vi "crio_FPGA_Stepper.vi"() -> ()   [LabVIEW 2019]
uses:
  <vilib>/rvi/Emulation/niFpgaSctlEmulationGetInTimedLoop.vi
  <vilib>/rvi/Emulation/niFpgaProcessEmulError.vi
  <vilib>/rvi/Emulation/niFpgaGetClockAttributes.vi
  <vilib>/rvi/Emulation/niFpgaEmulationReportErrorSimple.vi
  <vilib>/rvi/eio/common/nirviEmuTemplateMethod_errors.vi
  <vilib>/rvi/Emulation/niFpgaCriticalErrorInLSC.vi
  <vilib>/eio/EIONode/EIONode.xnode
panel:
  in  "Initial Position":i16=1
  in  "Position Control: Desired Positoin":i16=20000
  out "Controller Direction":bool
  out "Controller Enable":bool
  in  "Stepper Enable":bool
  in  "Manual Operation":bool
  in  "Rail soft limit":i16=10000
  in  "mSec to initialize a small push away from limit switch":u32=1 caption="mSec when hit limit"
  in  "mSec when hit limit":u32=100 caption="mSec to pause when hit limit"
  out "Platform Position":i16=20000
  out "Limit Switch":bool
  in  "stop":bool
  in  "Half Peirod (pulse 40MHz)":u32=10000 caption="Count(Tick) [Interval between step]"
  in  "Stepper Direction":bool
  # "1. Manual Control Mode: Turn on Manual Operation. Specify stepper direction. Hit enable to move.\n2. Auto Position Control Mode: Enter desired position. It will automatically go there.\n3. Whenever the platform hits the limit switch at the end it will reset position to 0.\n4. Rail's soft limit is only active under manual mode."
  # "Control Panel"
  # "20000 is about the limit"
  # "Every 10000 step is about 230mm,\nSo every step is about 2.3micron"
  # "High: towards limit switch,\nLow: towards NEMA"
  # "For debug"
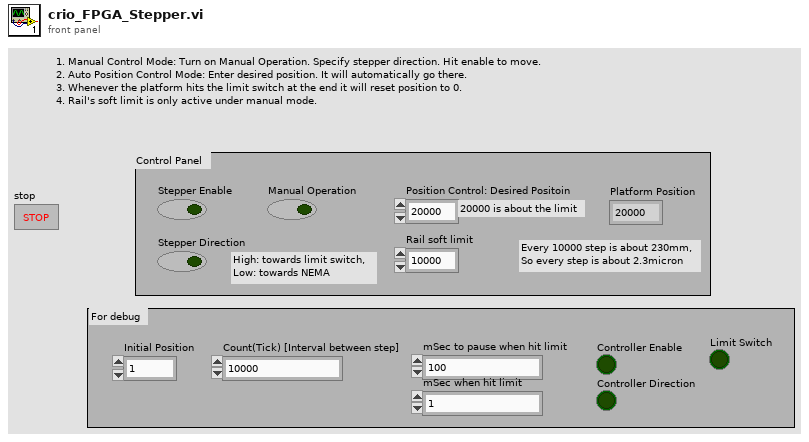
[diagram p1: front panel]
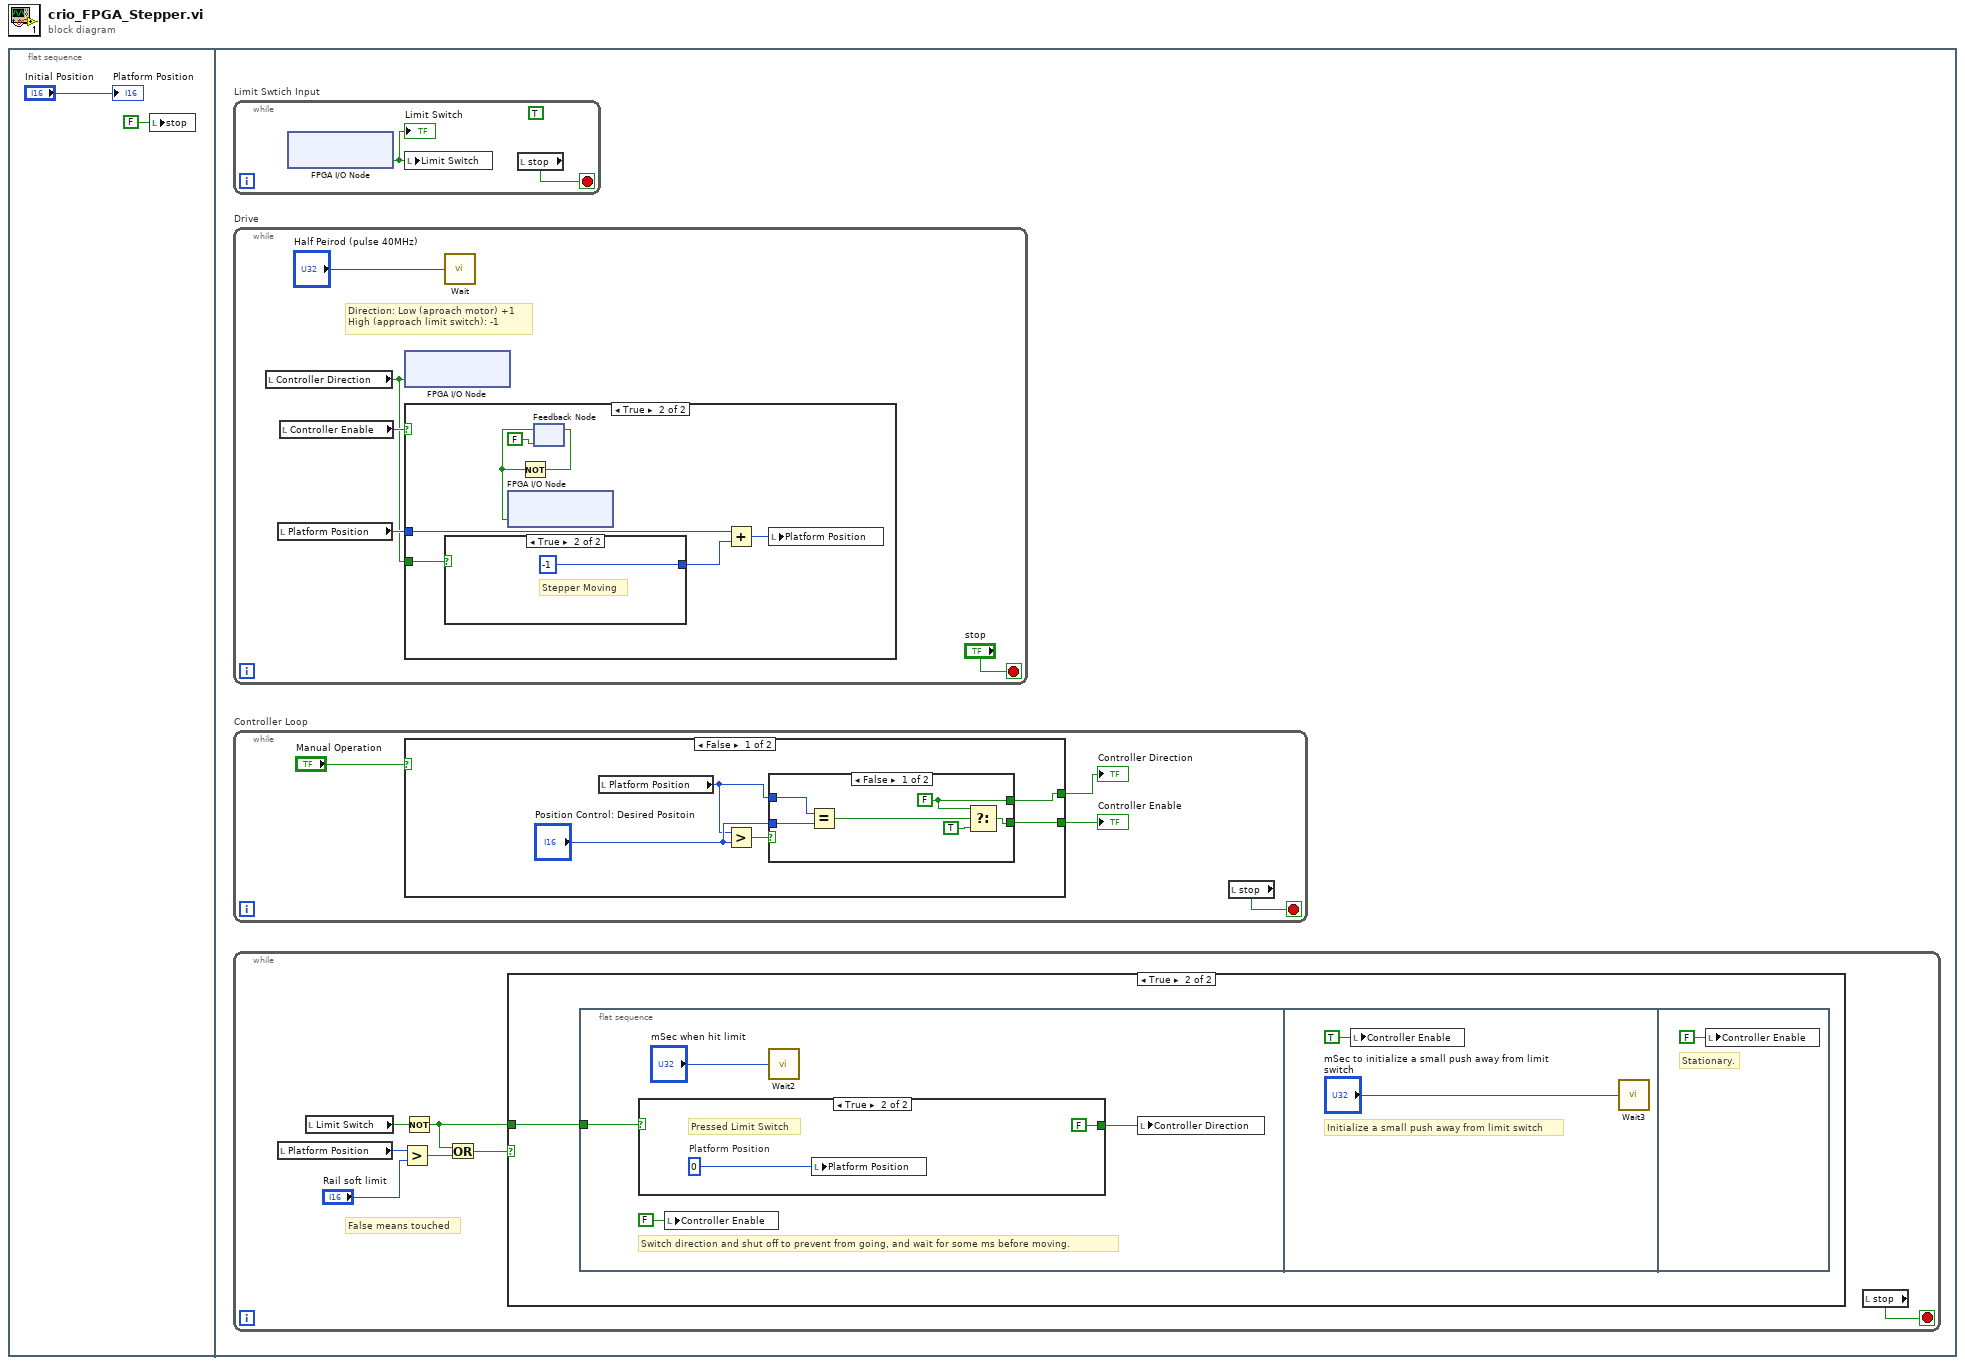
[diagram p0: block diagram]
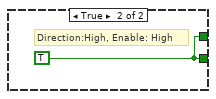
[diagram p2: hidden frame]
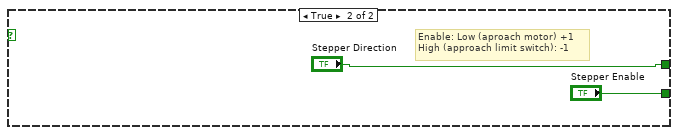
[diagram p3: hidden frame]
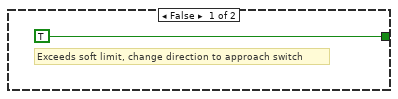
[diagram p5: hidden frame]
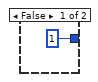
[diagram p7: hidden frame]
diagram:
  n1 = flat-sequence {
    frame #0 {
      n2 = local write "stop"(FALSE ("stop")) -> ()
      "Platform Position" <- "Initial Position"
    }
    frame #1 {
      n3 = while "Limit Swtich Input" {
        stop <- w39 stop-if-true
        (unwired) TRUE ("Mod8/DIO2")
        n4 = xnode "FPGA I/O Node"() -> ("Mod8/DIO2"=w40:bool)  [unwired: 1 in, 1 out]
        "Limit Switch" <- w40
        n5 = local write "Limit Switch"(w40) -> ()
        n6 = local read "stop"() -> (w39:bool)
      }
      n7 = while "Drive" {
        stop <- "stop" stop-if-true
        # "Direction: Low (aproach motor) +1\nHigh (approach limit switch): -1"
        n8 = local read "Controller Direction"() -> (w41:bool)
        n9 = local read "Platform Position"() -> (w43:i16)
        n10 = local read "Controller Enable"() -> (w42:bool)
        n11 = xnode "FPGA I/O Node"("Mod8/DIO4"=w41) -> ()  [unwired: 1 in, 1 out]
        n12 = case shown="True" w42 {
          tunnel: w41 -> [_ w49]
          tunnel: w43 -> [_ w46]
          frame False {
          }
          frame True {
            n13 = case shown="True" w49 {
              tunnel: [i16 1 i16 -1] -> w48
              frame False {
              }
              frame True {
                # "Stepper Moving"
              }
            }
            n14 = feedback #1(FALSE ("Connector0/DIO0")) -> (w50:bool)
            n15 = xnode "FPGA I/O Node"("Mod8/DIO3"=w50) -> ()  [unwired: 1 in, 1 out]
            n16 = Not(x=w50) -> (.not. x?=w51:bool)
            n17 = feedback-in #1(w51) -> ()
            n18 = Add(x=w46, y=w48) -> (x+y=w47:i16)
            n19 = local write "Platform Position"(w47) -> ()
          }
        }
        n20 = call "Wait"("Count(Ticks)"="Half Peirod (pulse 40MHz)") -> ()  [unwired: 1 out]
      }
      n21 = while "Controller Loop" {
        stop <- w6 stop-if-true
        n22 = case shown="False" "Manual Operation" {
          tunnel: [w10 "Stepper Enable"] -> w4
          tunnel: [w9 "Stepper Direction"] -> w3
          frame False {
            n23 = local read "Platform Position"() -> (w7:i16)
            n24 = Greater?(x=w7, y="Position Control: Desired Positoin") -> (0:w11:bool)
            n25 = case shown="False" w11 {
              tunnel: [w14 w18] -> w10
              tunnel: [w12 w18] -> w9
              tunnel: "Position Control: Desired Positoin" -> [w17 _]
              tunnel: w7 -> [w16 _]
              frame False {
                w12 = FALSE
                n26 = Equal?(x=w16, y=w17) -> (x = y?=w15:bool)
                n27 = Select(t=w12, s=w15, f=TRUE) -> (s? t:f=w14:bool)
              }
              frame True {
                w18 = TRUE
                # "Direction:High, Enable: High"
              }
            }
          }
          frame True {
            # "Enable: Low (aproach motor) +1\nHigh (approach limit switch): -1"
          }
        }
        "Controller Enable" <- w4
        "Controller Direction" <- w3
        n28 = local read "stop"() -> (w6:bool)
      }
      n29 = while {
        stop <- w27 stop-if-true
        # "False means touched"
        n30 = local read "Platform Position"() -> (w26:i16)
        n31 = local read "Limit Switch"() -> (w22:bool)
        n32 = Greater?(x=w26, y="Rail soft limit") -> (0:w24:bool)
        n33 = Not(x=w22) -> (.not. x?=w21:bool)
        n34 = Or(x=w21, y=w24) -> (x .or. y?=w23:bool)
        n35 = case shown="True" w23 {
          tunnel: w21 -> [_ w28]
          frame False {
            # "Do nothing"
          }
          frame True {
            n36 = flat-sequence {
              tunnel: w28 -> [w29]
              frame #0 {
                # "Switch direction and shut off to prevent from going, and wait for some ms before moving."
                n37 = case shown="True" w29 {
                  tunnel: [TRUE ("Stepper Direction") FALSE ("Stepper Direction")] -> w30
                  frame False {
                    # "Exceeds soft limit, change direction to approach switch"
                  }
                  frame True {
                    w35 = i16 0  # Platform Position
                    # "Pressed Limit Switch"
                    n38 = local write "Platform Position"(w35) -> ()
                  }
                }
                n39 = local write "Controller Enable"(FALSE ("Stepper Direction")) -> ()
                n40 = call "Wait2"("Count(mSec)"="mSec when hit limit") -> ()  [unwired: 1 out]
                n41 = local write "Controller Direction"(w30) -> ()
              }
              frame #1 {
                # "Initialize a small push away from limit switch"
                n42 = local write "Controller Enable"(TRUE ("Stepper Enable")) -> ()
                n43 = call "Wait3"("Count(mSec)"="mSec to initialize a small push away from limit switch") -> ()  [unwired: 1 out]
              }
              frame #2 {
                # "Stationary."
                n44 = local write "Controller Enable"(FALSE ("Stepper Enable")) -> ()
              }
            }
          }
        }
        n45 = local read "stop"() -> (w27:bool)
      }
    }
  }
